vi "Quick Usb Get Firmware Version.vi"(0 "hDevice":u32, 5 "MajorFirmwareVersion":u16, 7 "MinorFirmwareVersion":u16, 9 "BuildFirmwareVersion":u16, 11 "error in (no error)":errorcluster) -> (3 "function return":i32, 4 "hDevice out":u32, 6 "MajorFirmwareVersion out":u16, 8 "MinorFirmwareVersion out":u16, 10 "BuildFirmwareVersion out":u16, 15 "error out":errorcluster)   [LabVIEW 2011, in "QuickUSB.lvlib"]
doc: "QUSBLIB QRETURN QuickUsbGetFirmwareVersion(\n QHANDLE hDevice, \n PQWORD MajorFirmwareVersion,\n PQWORD MinorFirmwareVersion,\n PQWORD BuildFirmwareVersion\n);"
uses:
  QuickUSB.lvlib
  QuickUSB.dll
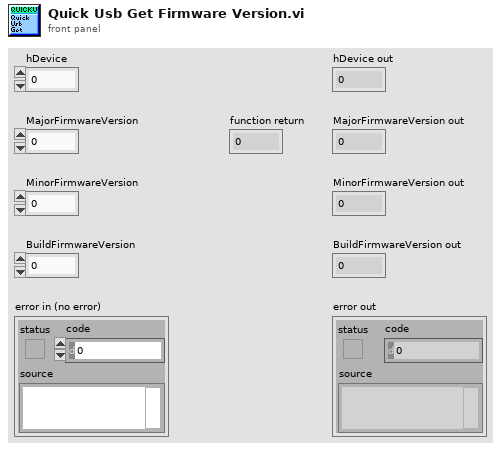
[diagram p1: front panel]
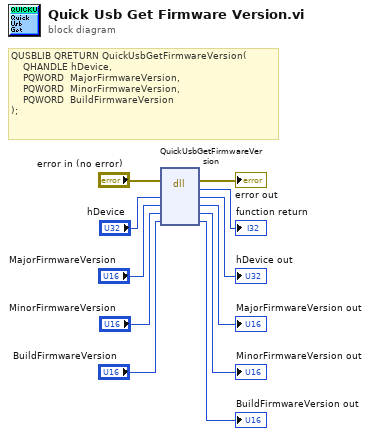
[diagram p0: block diagram]
diagram:
  # "QUSBLIB QRETURN QuickUsbGetFirmwareVersion(\n    QHANDLE hDevice, \n    PQWORD  MajorFirmwareVersion,\n    PQWORD  MinorFirmwareVersion,\n    PQWORD  BuildFirmwareVersion\n);"
  n1 = dll-call lib="C:/QuickUSB/QuickUSB.*" fn="QuickUsbGetFirmwareVersion"(error in="error in (no error)", "hDevice"="hDevice", "MajorFirmwareVersion"="MajorFirmwareVersion", "MinorFirmwareVersion"="MinorFirmwareVersion", "BuildFirmwareVersion"="BuildFirmwareVersion") -> (error out=→"error out":errorcluster, →"function return":i32, "hDevice"=→"hDevice out":u32, "MajorFirmwareVersion"=→"MajorFirmwareVersion out":u16, "MinorFirmwareVersion"=→"MinorFirmwareVersion out":u16, "BuildFirmwareVersion"=→"BuildFirmwareVersion out":u16)  [unwired: 2 in, 1 out]
